vi "WaveformAcqProcess.vi"(0 "Task in":refnum<class "WaveformTask.lvclass">, 1 "Buffers":T1, 11 "error in (no error)":errorcluster) -> ()   [LabVIEW 2015]
uses:
  <vilib>/NI/PowerElectronicsControl/BufferLogging/Buffers.ctl
  <vilib>/NI/PowerElectronicsControl/WaveformAcq/IFw_Addon/RT/WaveformTask.lvclass
  <vilib>/NI/PowerElectronicsControl/WaveformAcq/IFw_Addon/RT/ReadInterleaved.vi
  <vilib>/NI/PowerElectronicsControl/BufferLogging/BufferLogging.lvlib
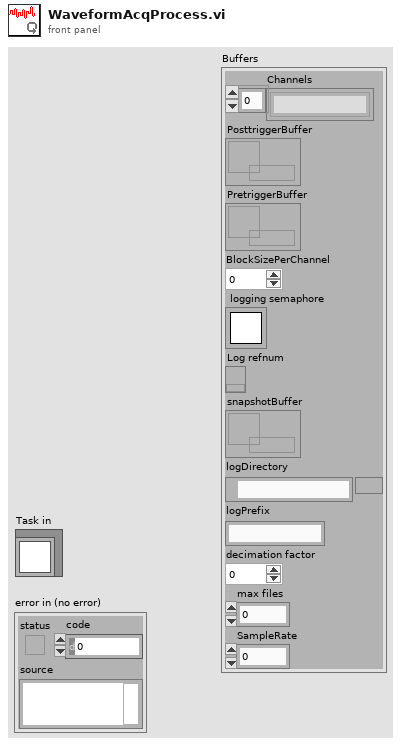
[diagram p1: front panel]
types:
  T1 = typedef "BufferLogging.lvlib/Buffers.ctl" = cluster{"Channels":string[], "PosttriggerBuffer":refnum<queue>, "PretriggerBuffer":refnum<queue>, "BlockSizePerChannel":i32, " logging semaphore":T2, "Log refnum":refnum<k34>, "snapshotBuffer":refnum<data-value>, "logDirectory":path, "logPrefix":string, "decimation factor":i32, "max files":i32, "SampleRate":dbl}
  T2 = typedef "Semaphore RefNum" = refnum<k1>
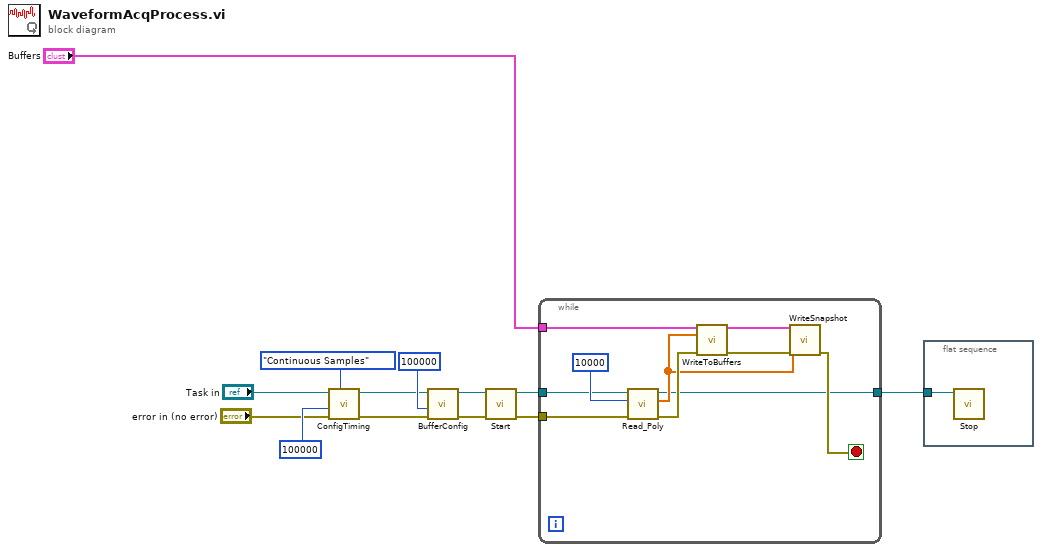
[diagram p0: block diagram]
diagram:
  n1 = call <vilib>:"ConfigTiming.vi"("Sample Mode"=enum16{"Finite Samples", "Continuous Samples"}."Continuous Samples", "error in (no error)"="error in (no error)", "Sample Rate"=u32 100000, "Task in"="Task in") -> ("error out"=w6:errorcluster, "Task out"=w5:refnum<class "WaveformTask.lvclass">)  [unwired: 5 in, 1 out]
  n2 = call <vilib>:"BufferConfig.vi"("error in (no error)"=w6, "Buffer Size [Samps per Chan]"=100000, "WaveformTask in"=w5) -> ("error out"=w9:errorcluster, "WaveformTask out"=w8:refnum<class "WaveformTask.lvclass">)  [unwired: 6 in, 1 out]
  n3 = call <vilib>:"Start.vi"("error in (no error)"=w9, "WaveformTask in"=w8) -> ("error out"=w11:errorcluster, "WaveformTask out"=w10:refnum<class "WaveformTask.lvclass">)  [unwired: 8 in]
  n4 = while {
    tunnel: w10 -> [w22]
    tunnel: "Buffers" -> [w17]
    tunnel: w11 -> [w21]
    tunnel: [w14] -> w12
    stop <- w15 stop-if-true
    n5 = call-poly <vilib>:"Read_Poly.vi"("error in"=w21, "Samps Read per Chan"=10000, "Task in"=w22) -> ("error out"=w18:errorcluster, "Data"=w16:sgl[], "Task out"=w14:refnum<class "WaveformTask.lvclass">)  [unwired: 5 in, 1 out]
    n6 = call <vilib>:"WriteToBuffers.vi"("Buffers in"=w17, "Data"=w16, "error in (no error)"=w18) -> ("Buffers out"=w19:T1, "error out"=w20:errorcluster)  [unwired: 11 in]
    n7 = call <vilib>:"WriteSnapshot.vi"("Buffers in"=w19, "Snapshot"=w16, "error in (no error)"=w20) -> ("error out"=w15:errorcluster)  [unwired: 11 in, 1 out]
  }
  n8 = flat-sequence {
    tunnel: w12 -> [w24]
    frame #0 {
      n9 = call <vilib>:"Stop.vi"("WaveformTask in"=w24) -> ()  [unwired: 9 in, 2 out]
    }
  }
